vi "Output_Algo.vi"(8 "error in":errorcluster, 9 "State":string, 10 "OutputCluster":T3={"Acknowledgement"={"Enqueuer"=refnum, "VIReference"=refnum, "VIName"=""}, "AllPartInfo"=[{"PartName"="", "NumberOfRacks"=0, "MeasurementIDsArray"=[], "MeasurementNamesArray"=[], "SpecValuesArray"=[]}], "PartInfo"={"PartName"="", "TotalCount"=0, "ReelCount"=0, "NumberOfRacks"=0, "MeasurementIDsArray"=[], "MeasurementNamesArray"=[], "SpecValuesArray"=[]}, "Result Cluster"={"Measurement Names Array"=[], "Pass-Fail Array"=[], "Measurement Values Array "=[], "Roi for overlay (Arrows) Array"=[], "Algo Type Array"=[], "Image Array"=[], "Clamp operations"=enum."Average Clamp", "  Search Direction "=[], "Images_Array_in"=[], "ResultPF"=FALSE, "Total Cluster Values"={"Total Fail"=0, "Total Pass"=0, "Total Count"=0}, "Reel Counter Cluster"={"Reel Fail"=0, "Reel Pass"=0, "Reel Count"=0}, "Tolerance  Array"=[], "Array of Cam Spec Control Bool"=[], "Control Pass Fail Array"=[], "Specification Pass Fail Array"=[], "Overlay Arrow Lines"=[], "Camera ID"=[], "Trigger count"=0, "Specification fail?"=FALSE}, "ErrorMessage"=""}, 11 "Private Data In":refnum<class "Algorithm.lvclass">) -> (0 "error out":errorcluster, 3 "Private Data Out":refnum<class "Algorithm.lvclass">)   [LabVIEW 2019, in "Algorithm.lvclass"]
uses:
  FrameworkOverrides/Algorithm.lvclass
  Rack Controller/Rack Controller Messages/Acknowledgement_RC Msg/Acknowledgement_RC Msg.lvclass
  Rack Controller/Rack Controller Messages/AllPartInfo_RC Msg/AllPartInfo_RC Msg.lvclass
  <vilib>/ActorFramework/Actor/Actor.lvclass
  Rack Controller/Rack Controller Messages/Part Info from Algo_RC Msg/Part Info from Algo_RC Msg.lvclass
  Rack Controller/Rack Controller Messages/Algorithm Result User Event_RC Msg/Algorithm Result User Event_RC Msg.lvclass
  Rack Controller/Rack Controller Messages/Error Message_RC Msg/Error Message_RC Msg.lvclass
  C:/Program Files/National Instruments/LabVIEW 2019/vi.lib/ActorFramework/Actor/Actor.lvclass
  <vilib>/ActorFramework/Message Enqueuer/Message Enqueuer.lvclass
  Common/Controls/AllPartInfo.ctl
  Common/Controls/Acknowledgement.ctl
  Controls/OutputCluster.ctl
  Controls/Result Cluster.ctl
  <vilib>/vision/Image Controls.llb/IMAQ Image.ctl
  Rack Controller/Controls/Result Cluster_RC.ctl
  Rack Controller/Rack Controller.lvclass
panel:
  in  "Algorithm Result Data":T1={"Measurement Values Array "=[0.1, 0.2], "Images Array"=[], "Result PF"=TRUE, "Production Count Details"={"Total Fail"=0, "Total Pass"=0, "Total Count"=0}, "Reel Count Details"={"Reel Fail"=0, "Reel Pass"=0, "Reel Count"=0}, "Control PF Array"=[TRUE, TRUE], "Specification PF Array"=[TRUE, TRUE], "Specification Fail?"=FALSE}
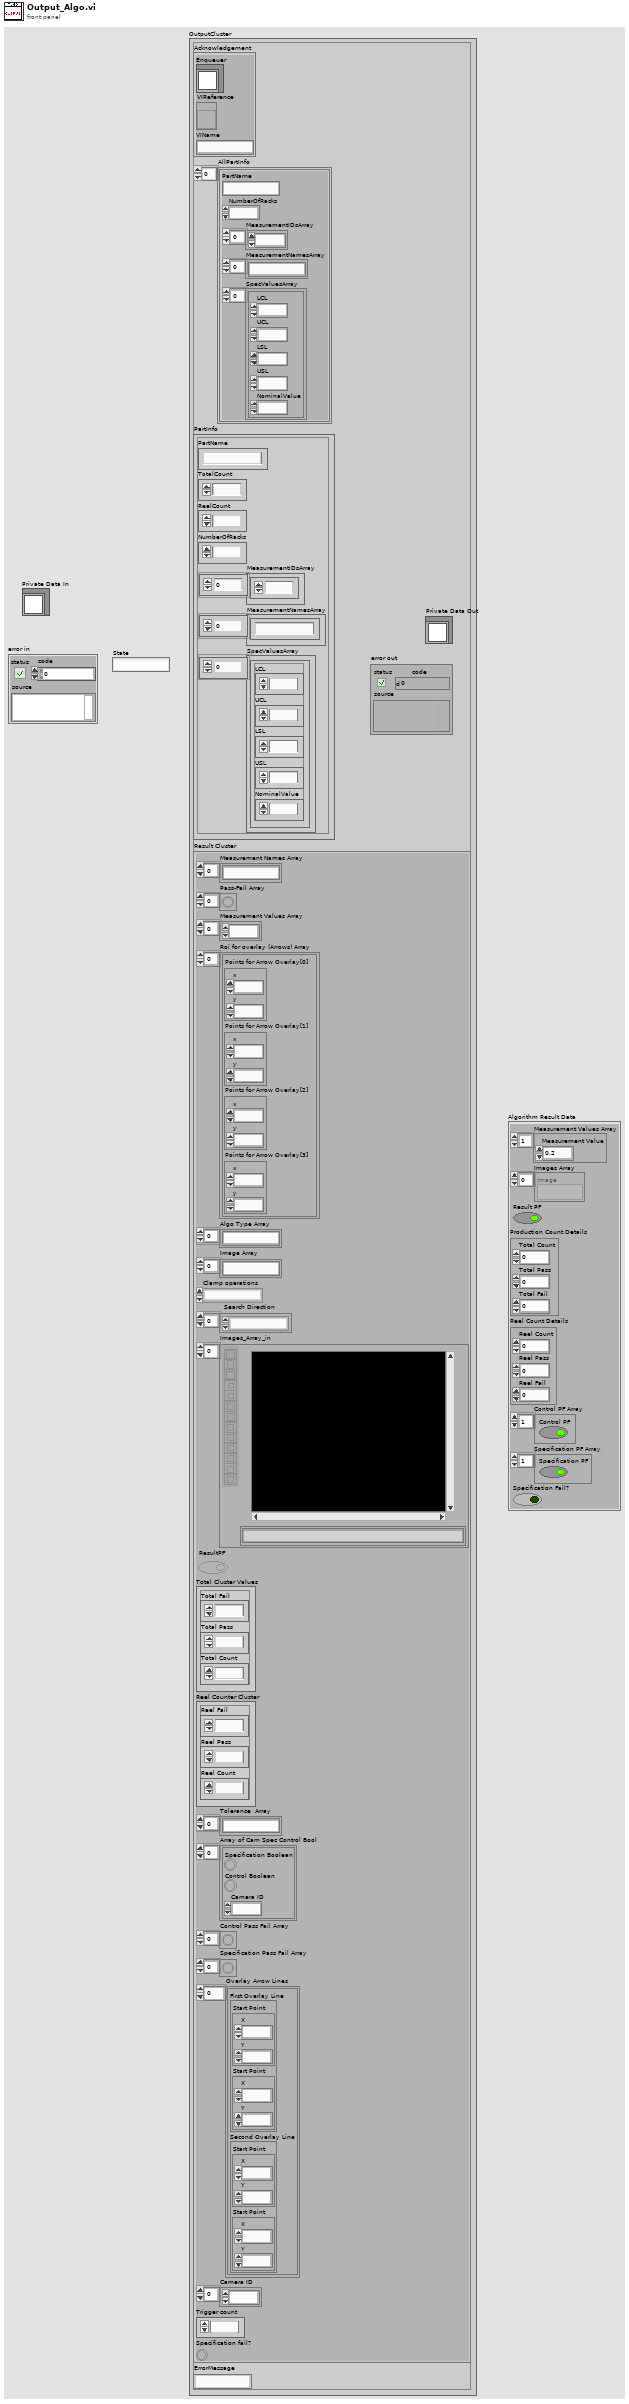
[diagram p1: front panel]
types:
  T1 = typedef "Rack Controller.lvclass/Result Cluster_RC.ctl" = cluster{"Measurement Values Array ":dbl[], "Images Array":T2[], "Result PF":bool, "Production Count Details":cluster{"Total Fail":u64, "Total Pass":u64, "Total Count":u64}, "Reel Count Details":cluster{"Reel Fail":u64, "Reel Pass":u64, "Reel Count":u64}, "Control PF Array":bool[], "Specification PF Array":bool[], "Specification Fail?":bool}
  T2 = typedef "IMAQ Image.ctl" = refnum<image>
  T3 = typedef "Algorithm.lvclass/OutputCluster.ctl" = cluster{"Acknowledgement":T4, "AllPartInfo":T5, "PartInfo":cluster{"PartName":string, "TotalCount":u64, "ReelCount":u64, "NumberOfRacks":u8, "MeasurementIDsArray":u16[], "MeasurementNamesArray":string[], "SpecValuesArray":cluster{"LCL":dbl, "UCL":dbl, "LSL":dbl, "USL":dbl, "NominalValue":dbl}[]}, "Result Cluster":T6, "ErrorMessage":string}
  T4 = typedef "Acknowledgement.ctl" = cluster{"Enqueuer":refnum<class "Message Enqueuer.lvclass">, "VIReference":refnum<vi>, "VIName":string}
  T5 = typedef "AllPartInfo.ctl" = cluster{"PartName":string, "NumberOfRacks":u8, "MeasurementIDsArray":u16[], "MeasurementNamesArray":string[], "SpecValuesArray":cluster{"LCL":dbl, "UCL":dbl, "LSL":dbl, "USL":dbl, "NominalValue":dbl}[]}[]
  T6 = typedef "Algorithm.lvclass/Result Cluster.ctl" = cluster{"Measurement Names Array":string[], "Pass-Fail Array":bool[], "Measurement Values Array ":dbl[], "Roi for overlay (Arrows) Array":cluster{"Points for Arrow Overlay[0]":cluster{"x":dbl, "y":dbl}, "Points for Arrow Overlay[1]":cluster{"x":dbl, "y":dbl}, "Points for Arrow Overlay[2]":cluster{"x":dbl, "y":dbl}, "Points for Arrow Overlay[3]":cluster{"x":dbl, "y":dbl}}[], "Algo Type Array":string[], "Image Array":string[], "Clamp operations":enum16{"Min Clamp", "Max Clamp", "Average Clamp"}, "  Search Direction ":enum16{"Left to Right", "Right to Left", "Top to Bottom", "Bottom to Top"}[], "Images_Array_in":T2[], "ResultPF":bool, "Total Cluster Values":cluster{"Total Fail":u64, "Total Pass":u64, "Total Count":u64}, "Reel Counter Cluster":cluster{"Reel Fail":u64, "Reel Pass":u64, "Reel Count":u64}, "Tolerance  Array":string[], "Array of Cam Spec Control Bool":cluster{"Specification Boolean":bool, "Control Boolean":bool, "Camera ID":i8}[], "Control Pass Fail Array":bool[], "Specification Pass Fail Array":bool[], "Overlay Arrow Lines":cluster{"First Overlay Line ":cluster{"Start Point":cluster{"X":sgl, "Y":sgl}, "Start Point":cluster{"X":sgl, "Y":sgl}}, "Second Overlay Line ":cluster{"Start Point":cluster{"X":sgl, "Y":sgl}, "Start Point":cluster{"X":sgl, "Y":sgl}}}[], "Camera ID":i8[], "Trigger count":i32, "Specification fail?":bool}
  T7 = cluster{"PartName":string, "MeasurementIDsArray":u16[], "MeasurementNamesArray":string[], "SpecValuesArray":cluster{"LCL":dbl, "UCL":dbl, "LSL":dbl, "USL":dbl, "NominalValue":dbl}[]}
  T8 = cluster{"Total Fail":u64, "Total Pass":u64, "Total Count":u64}
  T9 = cluster{"Reel Fail":u64, "Reel Pass":u64, "Reel Count":u64}
  T10 = cluster{"LCL":dbl, "UCL":dbl, "LSL":dbl, "USL":dbl, "NominalValue":dbl}[]
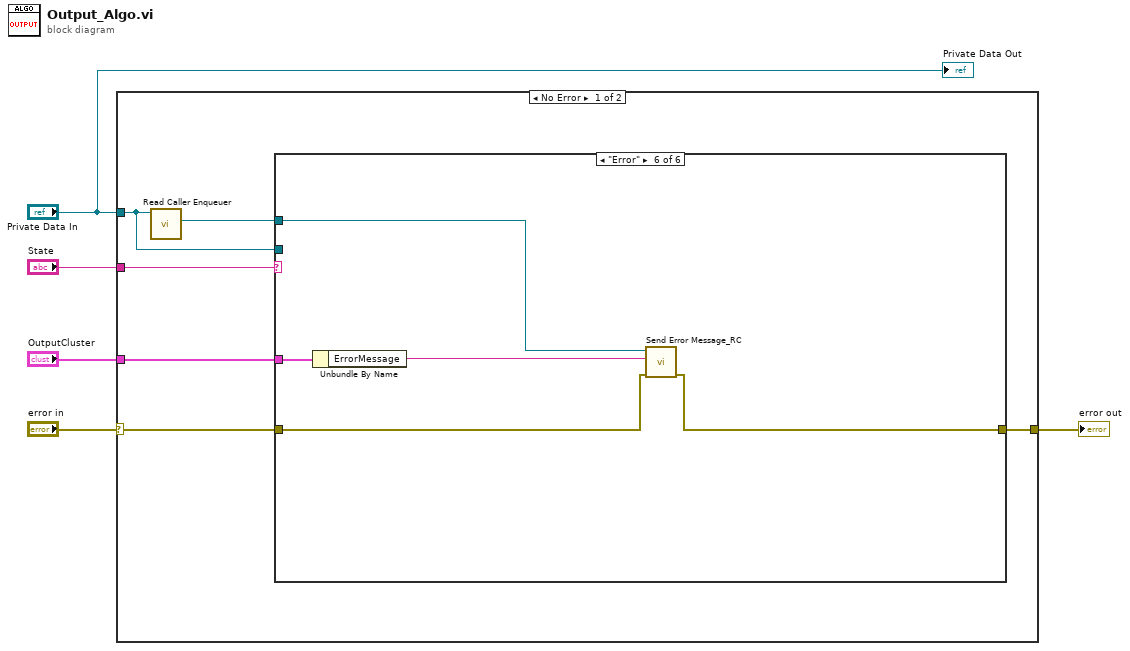
[diagram p0: block diagram]
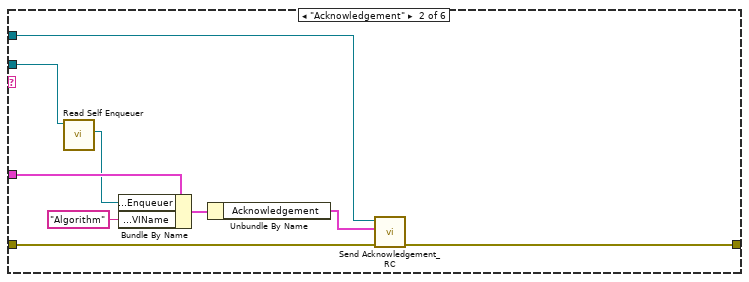
[diagram p3: hidden frame]
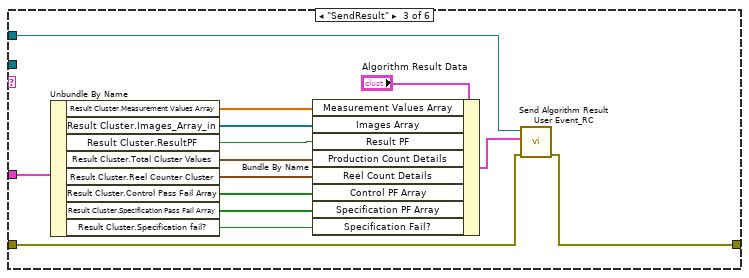
[diagram p4: hidden frame]
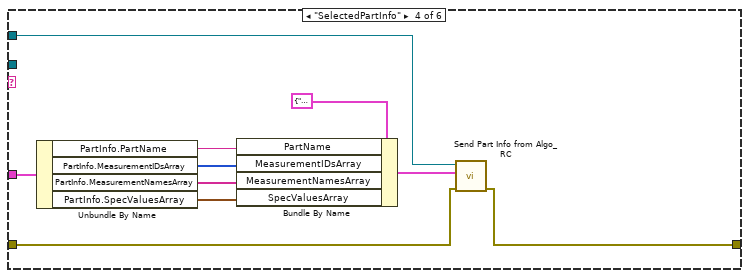
[diagram p5: hidden frame]
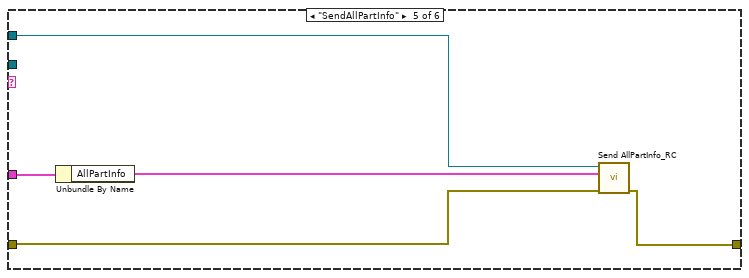
[diagram p6: hidden frame]
diagram:
  n1 = case shown="No Error" "error in" {
    selector: "error in" -> [w8 w56]
    tunnel: "OutputCluster" -> [w10 _]
    tunnel: "State" -> [w11 _]
    tunnel: "Private Data In" -> [w6 _]
    tunnel: [w9 w56] -> w2
    frame No Error {
      n2 = call <vilib>:"Read Caller Enqueuer.vi"("Actor"=w6) -> ("Caller Enqueuer"=w7:refnum<class "Message Enqueuer.lvclass">)  [unwired: 10 in]
      n3 = case shown="\"Error\"" w11 {
        tunnel: w7 -> [_ w19 w35 w42 w48 w53]
        tunnel: w10 -> [_ w18 w30 w45 w46 w55]
        tunnel: [w12 w20 w31 w36 w49 w51] -> w9
        tunnel: w8 -> [w12 w21 w32 w37 w47 w52]
        tunnel: w6 -> [_ w17 _ _ _ _]
        frame Default {
        }
        frame "Acknowledgement" {
          n4 = call <vilib>:"Read Self Enqueuer.vi"("Actor"=w17) -> ("Self Enqueuer"=w16:refnum<class "Message Enqueuer.lvclass">)  [unwired: 10 in]
          n5 = Bundle By Name(cluster=w18, "Acknowledgement.Enqueuer"=w16, "Acknowledgement.VIName"="Algorithm") -> (w14:T3)
          n6 = Unbundle By Name(w14) -> ("Acknowledgement"=w13:T4)
          n7 = call "Send Acknowledgement_RC.vi"("error in (no error)"=w21, "Acknowledgement_RC"=w13, "Message Enqueuer"=w19) -> ("error out"=w20:errorcluster)  [unwired: 7 in, 1 out]
        }
        frame "SendResult" {
          n8 = Unbundle By Name(w30) -> ("Result Cluster.Measurement Values Array"=w25:dbl[], "Result Cluster.Images_Array_in"=w29:T2[], "Result Cluster.ResultPF"=w26:bool, "Result Cluster.Total Cluster Values"=w28:T8, "Result Cluster.Reel Counter Cluster"=w27:T9, "Result Cluster.Control Pass Fail Array"=w24:bool[], "Result Cluster.Specification Pass Fail Array"=w23:bool[], "Result Cluster.Specification fail?"=w22:bool)
          n9 = Bundle By Name(cluster="Algorithm Result Data", "Measurement Values Array"=w25, "Images Array"=w29, "Result PF"=w26, "Production Count Details"=w28, "Reel Count Details"=w27, "Control PF Array"=w24, "Specification PF Array"=w23, "Specification Fail?"=w22) -> (w33:T1)
          n10 = call "Send Algorithm Result User Event_RC.vi"("error in (no error)"=w32, "Algorithm Result Data"=w33, "Message Enqueuer"=w35) -> ("error out"=w31:errorcluster)  [unwired: 7 in, 1 out]
        }
        frame "SelectedPartInfo" {
          n11 = Unbundle By Name(w45) -> ("PartInfo.PartName"=w41:string, "PartInfo.MeasurementIDsArray"=w40:u16[], "PartInfo.MeasurementNamesArray"=w39:string[], "PartInfo.SpecValuesArray"=w38:T10)
          n12 = Bundle By Name(cluster=T7 {"PartName"="", "MeasurementIDsArray"=[], "MeasurementNamesArray"=[], "SpecValuesArray"=[]} ("PartInfo"), "PartName"=w41, "MeasurementIDsArray"=w40, "MeasurementNamesArray"=w39, "SpecValuesArray"=w38) -> (w43:T7)
          n13 = call "Send Part Info from Algo_RC.vi"("error in (no error)"=w37, "PartInfo"=w43, "Message Enqueuer"=w42) -> ("error out"=w36:errorcluster)  [unwired: 7 in, 1 out]
        }
        frame "SendAllPartInfo" {
          n14 = Unbundle By Name(w46) -> ("AllPartInfo"=w50:T5)
          n15 = call "Send AllPartInfo_RC.vi"("error in (no error)"=w47, "AllPartInfo"=w50, "Message Enqueuer"=w48) -> ("error out"=w49:errorcluster)  [unwired: 7 in, 1 out]
        }
        frame "Error" {
          n16 = Unbundle By Name(w55) -> ("ErrorMessage"=w54:string)
          n17 = call "Send Error Message_RC.vi"("error in (no error)"=w52, "Error Message_RC"=w54, "Message Enqueuer"=w53) -> ("error out"=w51:errorcluster)  [unwired: 7 in, 1 out]
        }
      }
    }
    frame Error {
    }
  }
  "error out" <- w2
  "Private Data Out" <- "Private Data In"
